vi "Configure Output.vi"(7 "Enable Output (T: Enable)":bool=TRUE, 8 "error in (no error)":errorcluster, 9 "Voltage Level (0.0 V)":dbl format="%.2g", 10 "Channel (1: Channel 1)":i32(ring)=1 items=["Channel 1"=1, "Channel 2"=2], 11 "VISA resource name":refnum<visa-resource-name>) -> (0 "error out":errorcluster, 3 "VISA resource name out":refnum<visa-resource-name>)   [LabVIEW 2024]
doc: "Configures output voltage level, channel, and enables or disables the output of the power supply."
uses:
  <instrlib>/Zatez Kopper/Zatez Kopper.lvlib
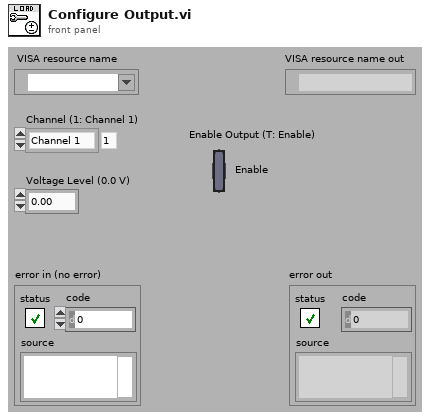
[diagram p1: front panel]
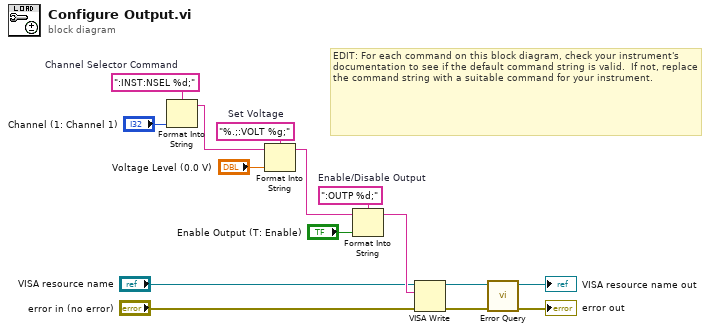
[diagram p0: block diagram]
diagram:
  w10 = ":OUTP %d;"  # Enable/Disable Output
  w1 = ":INST:NSEL %d;"  # Channel Selector Command
  w11 = "%.;:VOLT %g;"  # Set Voltage
  # "EDIT: For each command on this block diagram, check your instrument's documentation to see if the default command string is valid.  If not, replace the command string with a suitable command for your instrument."
  n1 = Format Into String(format string=w1, "Channel (1: Channel 1)") -> (resulting string=w5:string)  [unwired: 2 in, 1 out]
  n2 = Format Into String(format string=w11, initial string=w5, "Voltage Level (0.0 V)") -> (resulting string=w4:string)  [unwired: 1 in, 1 out]
  n3 = Format Into String(format string=w10, initial string=w4, "Enable Output (T: Enable)") -> (resulting string=w7:string)  [unwired: 1 in, 1 out]
  n4 = VISA Write(VISA resource name="VISA resource name", write buffer=w7, error in (no error)="error in (no error)") -> (VISA resource name out=w9:refnum<visa-resource-name>, error out=w8:errorcluster)  [unwired: 1 out]
  n5 = call <instrlib>:"Error Query.vi"("error in (no error)"=w8, "VISA resource name"=w9) -> ("error out"=→"error out":errorcluster, "VISA resource name out"=→"VISA resource name out":refnum<visa-resource-name>)  [unwired: 6 in, 2 out]
